vi "DelayGenerator-StaticBaseline.vi"(2 "site_info":T3 {"longitude" format="%_10g"; "latitude" format="%_10g"}, 3 "Time Stamp":timestamp, 5 "Baseline":T2 {"Up" format="%.6g"; "North" format="%.6g"; "East" format="%.6g"}, 7 "dt":dbl[unit]=66.131, 8 "cat_entry":T1 {"dec" format="%.6g"; "ra" format="%.6g"}, 9 "error in (no error)":errorcluster caption="error out") -> (0 "Delay":dbl[unit], 1 "Delay Rate":dbl[unit], 6 "error out":errorcluster)   [LabVIEW 2009]
uses:
  Controls/SiteInformation.ctl
  Controls/Baseline.ctl
  Controls/StarAstrometricEntry.ctl
  <vilib>/Analysis/baseanly.llb/Real Dot Product.vi
  <vilib>/Analysis/NI_AALBase.lvlib
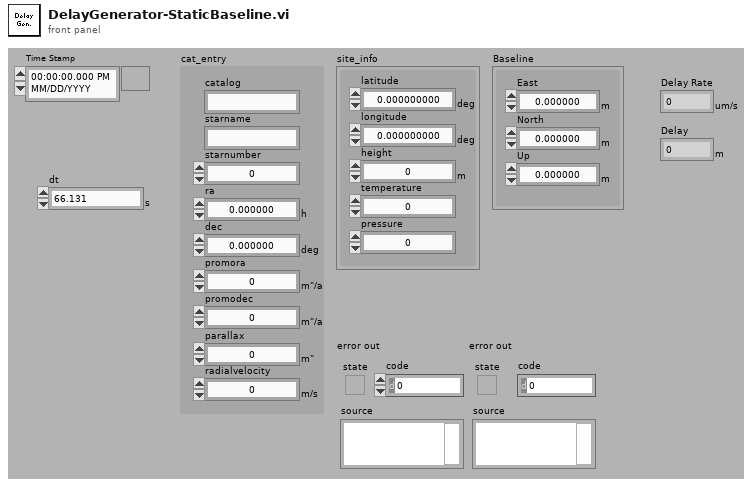
[diagram p1: front panel]
types:
  T1 = typedef "StarAstrometricEntry.ctl" = cluster{"catalog":string, "starname":string, "starnumber":i32, "ra":dbl[unit], "dec":dbl[unit], "promora":dbl[unit], "promodec":dbl[unit], "parallax":dbl[unit], "radialvelocity":dbl[unit]}
  T2 = typedef "Baseline.ctl" = cluster{"East":dbl[unit], "North":dbl[unit], "Up":dbl[unit]}
  T3 = typedef "SiteInformation.ctl" = cluster{"latitude":dbl[unit], "longitude":dbl[unit], "height":dbl[unit], "temperature":dbl, "pressure":dbl}
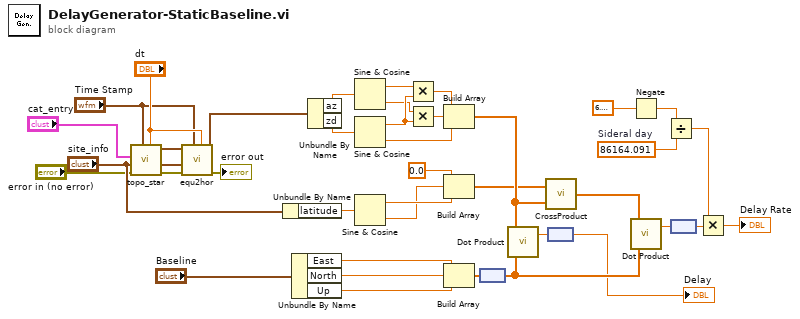
[diagram p0: block diagram]
diagram:
  w7 = dbl[unit] 86164.091  # Sideral day
  n1 = call "topo_star.vi"("deltat (TT-UT1)"="dt", "TimeStamp [UT1]"="Time Stamp", "error in (no error)"="error in (no error)", "on_surface"="site_info", "cat_entry"="cat_entry") -> ("error out"=w12:errorcluster, "ra/dec"=w14:cluster{"ra":dbl[unit], "dec":dbl[unit]})  [unwired: 3 in]
  n2 = call "equ2hor.vi"("deltat [TT-UT1]"="dt", "TimeStamp [UT1]"="Time Stamp", "error in (no error)"=w12, "on_surface"="site_info", "ra/dec"=w14) -> ("error out"=→"error out":errorcluster, "az/zd"=w11:cluster{"az":dbl[unit], "zd":dbl[unit]})  [unwired: 2 in, 1 out]
  n3 = Unbundle By Name("site_info") -> ("latitude"=w34:dbl[unit])
  n4 = Unbundle By Name("Baseline") -> ("East"=w21:dbl[unit], "North"=w20:dbl[unit], "Up"=w22:dbl[unit])
  n5 = Unbundle By Name(w11) -> ("az"=w31:dbl[unit], "zd"=w24:dbl[unit])
  n6 = Sine & Cosine(0:w31) -> (1:w26:dbl, 2:w25:dbl)
  n7 = Sine & Cosine(0:w24) -> (1:w27:dbl, 2:w30:dbl)
  n8 = Sine & Cosine(0:w34) -> (1:w10:dbl, 2:w9:dbl)
  n9 = Multiply(x=w26, y=w27) -> (x*y=w28:dbl)
  n10 = Multiply(x=w25, y=w27) -> (x*y=w29:dbl)
  n11 = Build Array(w28, w29, w30) -> (w8:dbl[])
  n12 = Build Array(0.0 ("élément"), w9, w10) -> (w4:dbl[])
  n13 = Build Array(w21, w20, w22) -> (w19:dbl[unit][])
  n14 = node(w19) -> (w38:dbl[])
  n15 = call-poly <vilib>:"Dot Product.vi"("Y Vector"=w38, "X Vector"=w8) -> ("X * Y"=w23:dbl)  [unwired: 1 out]
  n16 = call "CrossProduct.vi"("V2"=w8, "V1"=w4) -> ("V1^V2"=w37:dbl[])
  n17 = node(w23) -> (→"Delay":dbl[unit])
  n18 = Negate(x=6.283185307179586) -> (-x=w2:dbl)
  n19 = call-poly <vilib>:"Dot Product.vi"("Y Vector"=w38, "X Vector"=w37) -> ("X * Y"=w36:dbl)  [unwired: 1 out]
  n20 = Divide(x=w2, y=w7) -> (x/y=w6:dbl[unit])
  n21 = node(w36) -> (w39:dbl[unit])
  n22 = Multiply(x=w6, y=w39) -> (x*y=→"Delay Rate":dbl[unit])
